vi "GetDisplacementProperties.vi"(11 "channel properties":T2[](array[typedef])) -> (3 "tdms properties":T1[](array[typedef]))   [LabVIEW 2017, in "Tdms.lvlib"]
uses:
  <vilib>/addons/InsightCM/Utilities/Tdms/Tdms.lvlib
  <vilib>/addons/InsightCM/MessageBus/Base/controls/KeyValuePair.ctl
  <vilib>/addons/InsightCM/Utilities/Tdms/controls/Property.ctl
  <vilib>/addons/InsightCM/Utilities/PropertyHelpers/PropertyHelpers.lvlib
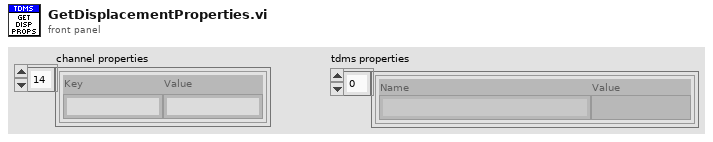
[diagram p1: front panel]
types:
  T1 = typedef "Tdms.lvlib/Property.ctl" = cluster{"Name":string, "Value":variant}
  T2 = typedef "KeyValuePair.ctl" = cluster{"Key":string, "Value":string}
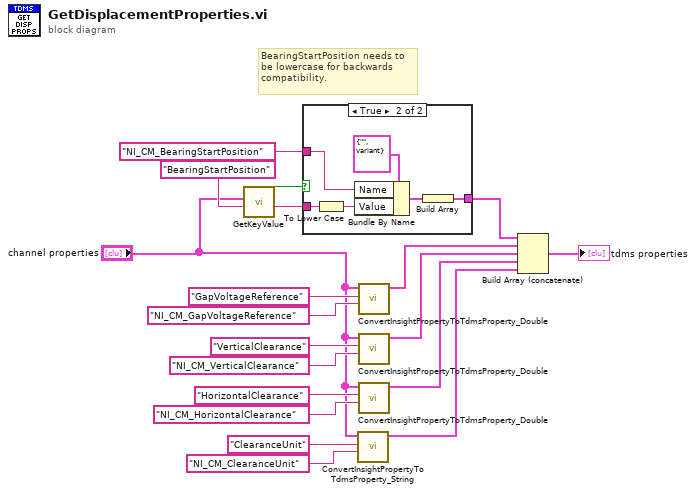
[diagram p0: block diagram]
diagram:
  # "BearingStartPosition needs to\nbe lowercase for backwards\ncompatibility."
  n1 = call <vilib>:"GetKeyValue.vi"("key"="BearingStartPosition" ("Name"), "key value pairs"="channel properties") -> ("value"=w6:string, "found"=w5:bool)  [unwired: 7 in, 1 out]
  n2 = case shown="True" w5 {
    tunnel: w6 -> [_ w21]
    tunnel: [_ w23] -> w2
    tunnel: "NI_CM_BearingStartPosition" ("Name") -> [_ w22]
    frame False {
    }
    frame True {
      n3 = To Lower Case(string=w21) -> (all lower case string=w20:string)
      n4 = Bundle By Name(cluster=T1 {"Name"="", "Value"=variant} ("Property"), "Name"=w22, "Value"=w20) -> (w24:T1)
      n5 = Build Array(w24) -> (w23:T1[])
    }
  }
  n6 = call <vilib>:"ConvertInsightPropertyToTdmsProperty_String.vi"("Tdms Property Name"="NI_CM_ClearanceUnit" ("Name"), "Insight Property Name"="ClearanceUnit" ("Name"), "Insight Properties"="channel properties") -> ("Tdms Properties"=w8:T1[])  [unwired: 8 in]
  n7 = call <vilib>:"ConvertInsightPropertyToTdmsProperty_Double.vi"("Tdms Property Name"="NI_CM_GapVoltageReference" ("Name"), "Insight Property Name"="GapVoltageReference" ("Name"), "Insight Properties"="channel properties") -> ("Tdms Properties"=w11:T1[])  [unwired: 8 in]
  n8 = call <vilib>:"ConvertInsightPropertyToTdmsProperty_Double.vi"("Tdms Property Name"="NI_CM_VerticalClearance" ("Name"), "Insight Property Name"="VerticalClearance" ("Name"), "Insight Properties"="channel properties") -> ("Tdms Properties"=w10:T1[])  [unwired: 8 in]
  n9 = call <vilib>:"ConvertInsightPropertyToTdmsProperty_Double.vi"("Tdms Property Name"="NI_CM_HorizontalClearance" ("Name"), "Insight Property Name"="HorizontalClearance" ("Name"), "Insight Properties"="channel properties") -> ("Tdms Properties"=w9:T1[])  [unwired: 8 in]
  n10 = Build Array (concatenate)(w2, w11, w10, w9, w8) -> (→"tdms properties":T1[])
